vi "HSV2RGB.vi"(3 "V":dbl, 4 "S":dbl, 5 "H":dbl) -> (0 "B":u8, 1 "G":u8, 2 "R":u8)   [LabVIEW 2020]
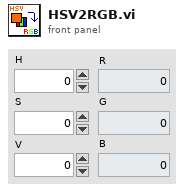
[diagram p1: front panel]
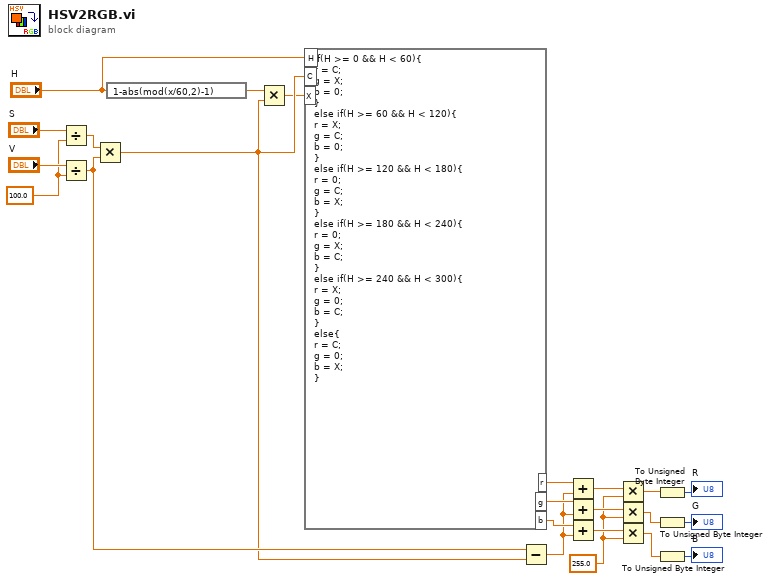
[diagram p0: block diagram]
diagram:
  w7 = 255.0
  w21 = 100.0
  n1 = Divide(x="S", y=w21) -> (x/y=w20:dbl)
  n2 = Divide(x="V", y=w21) -> (x/y=w18:dbl)
  n3 = Multiply(x=w20, y=w18) -> (x*y=w16:dbl)
  n4 = expression code="1-abs(mod(x/60,2)-1)"("H") -> (w19:dbl)
  n5 = Multiply(x=w19, y=w16) -> (x*y=w15:dbl)
  n6 = formula code="if(H >= 0 && H < 60){\nr = C;\ng = X;\nb = 0;\n}\nelse if(H >= 60 && H < 120){\nr = X;\ng = C;\nb = 0;\n}\nelse if(H >= 120 && H < 180){\nr = 0;\ng = C;\nb = X;\n}\nelse if(H >= 180 && H < 240){\nr = 0;\ng = X;\nb = C;\n}\nelse if(H >= 240 && H < 300){\nr = X;\ng = 0;\nb = C;\n}\nelse{\nr = C;\ng = 0;\nb = X;\n}"("H"="H", "C"=w16, "X"=w15) -> ("r"=w14:dbl, "g"=w13:dbl, "b"=w12:dbl)
  n7 = Subtract(x=w18, y=w16) -> (x-y=w11:dbl)
  n8 = Add(x=w14, y=w11) -> (x+y=w10:dbl)
  n9 = Add(x=w13, y=w11) -> (x+y=w9:dbl)
  n10 = Add(x=w12, y=w11) -> (x+y=w8:dbl)
  n11 = Multiply(x=w10, y=w7) -> (x*y=w3:dbl)
  n12 = Multiply(x=w9, y=w7) -> (x*y=w2:dbl)
  n13 = Multiply(x=w8, y=w7) -> (x*y=w1:dbl)
  n14 = To Unsigned Byte Integer(number=w3) -> (unsigned 8bit integer=→"R":u8)
  n15 = To Unsigned Byte Integer(number=w2) -> (unsigned 8bit integer=→"G":u8)
  n16 = To Unsigned Byte Integer(number=w1) -> (unsigned 8bit integer=→"B":u8)
